vi "ConfigInstr.vi"(6 "InstrumentName":string, 7 "VisaRessIn":refnum<visa-resource-name>, 8 "error in (no error)":errorcluster caption="entrée d'erreur (pas d'erreur)", 9 "FirstClassInst":bool, 10 "Function":string, 11 "GenData In":refnum<class "SymphonyCCD.lvclass"> caption="DNL_LabVIEW Object in") -> (0 "error out":errorcluster caption="sortie d'erreur", 3 "GenData Out":refnum<class "SymphonyCCD.lvclass"> caption="DNL_LabVIEW Object out")   [LabVIEW 2019, in "SymphonyCCD.lvclass"]
uses:
  SymphonyCCD.lvclass
  C:/Programmes Labview/LabScanV1A/DevicesClass/BaseDevice/BaseDevice.lvclass
  SymphonyCCD_Func.ctl
  SymphonyCCD.lvclass/SymphonyCCD.ctl
  BaseDevice/BaseDevice.lvclass/BaseDevice.ctl
  BaseDevice/Accessor/SetShowInstrNm.vi
  BaseDevice/Accessor/SetSaveArrVarPar.vi
  BaseDevice/Accessor/SetInstrParam.vi
panel:
  in  "Class_Func":T1
  out "VisaRessOut":refnum<visa-resource-name>
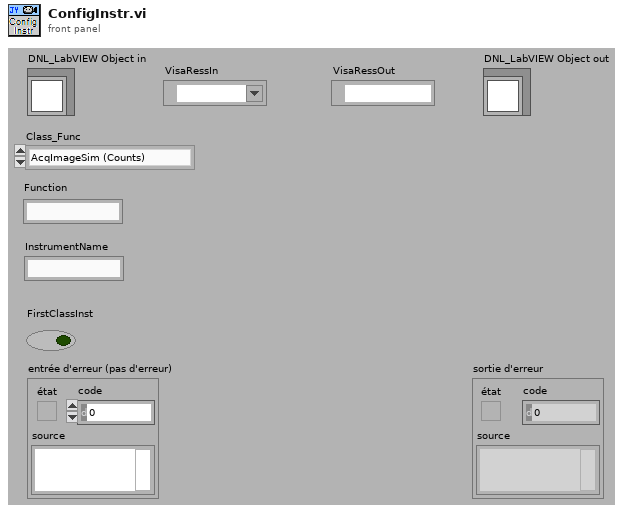
[diagram p1: front panel]
types:
  T1 = typedef "SymphonyCCD.lvclass/SymphonyCCD_Func.ctl" = enum16{"AcqImageSim (Counts)", "AcqImage (Counts)"}
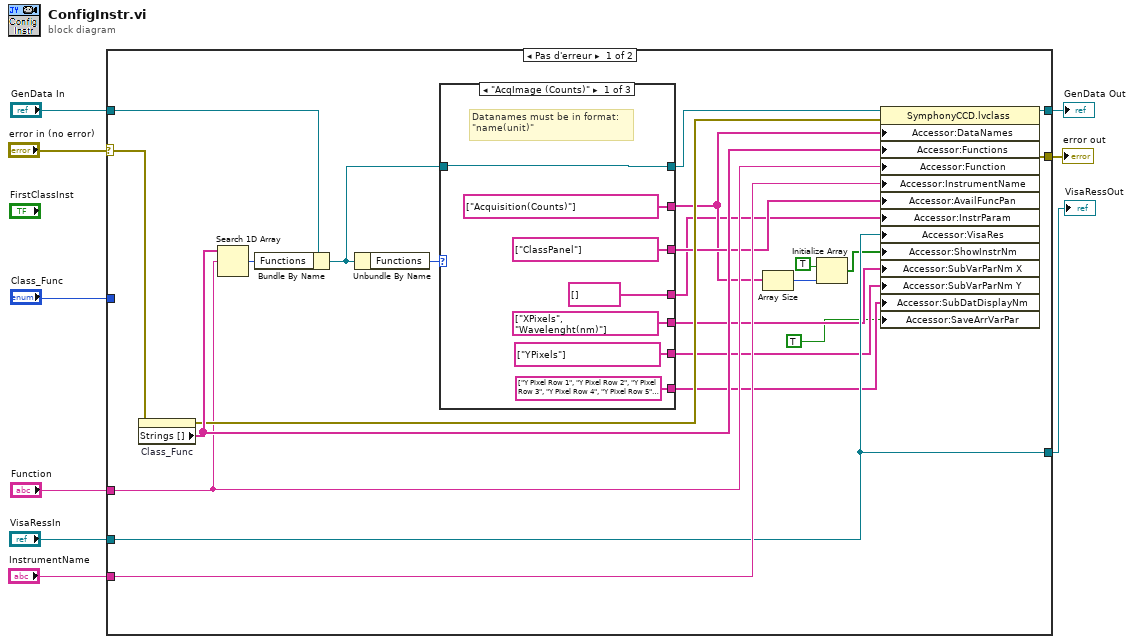
[diagram p0: block diagram]
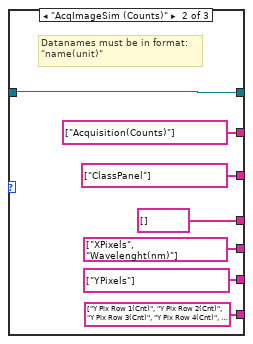
[diagram p2: hidden frame]
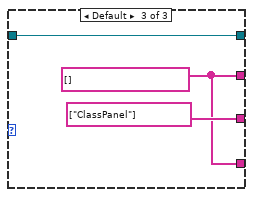
[diagram p3: hidden frame]
diagram:
  n1 = case shown="Pas d'erreur" "error in (no error)" {
    selector: "error in (no error)" -> [w26 w51]
    tunnel: [w32 w51] -> w8
    tunnel: "GenData In" -> [w27 w50]
    tunnel: [w31 w50] -> w6
    tunnel: "Class_Func" -> [_ _]
    tunnel: "Function" -> [w22 _]
    tunnel: "InstrumentName" -> [w21 _]
    tunnel: "VisaRessIn" -> [w19 _]
    tunnel: [w19 _] -> w1
    frame No Error {
      n2 = property on="Class_Func" class="Énum (strict)"(error in=w26) -> (error out=w25:errorcluster, "Strings []"=w29:string[])  [unwired: 1 in, 1 out]
      n3 = Search 1D Array(1D array=w29, element=w22) -> (index of element=w28:i32)  [unwired: 1 in]
      n4 = Bundle By Name(cluster=w27, "Functions"=w28) -> (w24:refnum<class "SymphonyCCD.lvclass">)
      n5 = Unbundle By Name(w24) -> ("Functions"=w30:T1)
      n6 = case shown="\"AcqImage (Counts)\"" w30 {
        tunnel: [string[] ["Acquisition(Counts)"] string[] ["Acquisition(Counts)"] w47] -> w16
        tunnel: w24 -> [w39 w46 w49]
        tunnel: [w39 w46 w49] -> w23
        tunnel: [string[] ["ClassPanel"] string[] ["ClassPanel"] string[] ["ClassPanel"]] -> w20
        tunnel: [string[] [] string[] [] w47] -> w14
        tunnel: [string[] ["XPixels", "Wavelenght(nm)"] string[] ["XPixels", "Wavelenght(nm)"] _] -> w13
        tunnel: [string[] ["YPixels"] string[] ["YPixels"] _] -> w12
        tunnel: [string[] ["Y Pixel Row 1", "Y Pixel Row 2", "Y Pixel Row 3", "Y Pixel Row 4", "Y Pixel Row 5", "Y Pixel Row 6", "Y Pixel Row 7", "Y Pixel Row 8", "Y Pixel Row 9", "Y Pixel Row 10", "Y Pixel Row 11", "Y Pixel Row 12", "Y Pixel Row 13", "Y Pixel Row 14", "Y Pixel Row 15", "Y Pixel Row 16", "Y Pixel Row 17", "Y Pixel Row 18", "Y Pixel Row 19", "Y Pixel Row 20", "Y Pixel Row 21", "Y Pixel Row 22", "Y Pixel Row 23", "Y Pixel Row 24", "Y Pixel Row 25", "Y Pixel Row 26", "Y Pixel Row 27", "Y Pixel Row 28", "Y Pixel Row 29", "Y Pixel Row 30", "Y Pixel Row 31", "Y Pixel Row 32", "Y Pixel Row 33", "Y Pixel Row 34", "Y Pixel Row 35", "Y Pixel Row 36", "Y Pixel Row 37", "Y Pixel Row 38", "Y Pixel Row 39", "Y Pixel Row 40", "Y Pixel Row 41", "Y Pixel Row 42", "Y Pixel Row 43", "Y Pixel Row 44", "Y Pixel Row 45", "Y Pixel Row 46", "Y Pixel Row 47", "Y Pixel Row 48", "Y Pixel Row 49", "Y Pixel Row 50", "Y Pixel Row 51", "Y Pixel Row 52", "Y Pixel Row 53", "Y Pixel Row 54", "Y Pixel Row 55", "Y Pixel Row 56", "Y Pixel Row 57", "Y Pixel Row 58", "Y Pixel Row 59", "Y Pixel Row 60", "Y Pixel Row 61", "Y Pixel Row 62", "Y Pixel Row 63", "Y Pixel Row 64", "Y Pixel Row 65", "Y Pixel Row 66", "Y Pixel Row 67", "Y Pixel Row 68", "Y Pixel Row 69", "Y Pixel Row 70", "Y Pixel Row 71", "Y Pixel Row 72", "Y Pixel Row 73", "Y Pixel Row 74", "Y Pixel Row 75", "Y Pixel Row 76", "Y Pixel Row 77", "Y Pixel Row 78", "Y Pixel Row 79", "Y Pixel Row 80", "Y Pixel Row 81", "Y Pixel Row 82", "Y Pixel Row 83", "Y Pixel Row 84", "Y Pixel Row 85", "Y Pixel Row 86", "Y Pixel Row 87", "Y Pixel Row 88", "Y Pixel Row 89", "Y Pixel Row 90", "Y Pixel Row 91", "Y Pixel Row 92", "Y Pixel Row 93", "Y Pixel Row 94", "Y Pixel Row 95", "Y Pixel Row 96", "Y Pixel Row 97", "Y Pixel Row 98", "Y Pixel Row 99", "Y Pixel Row 100", "Y Pixel Row 101", "Y Pixel Row 102", "Y Pixel Row 103", "Y Pixel Row 104", "Y Pixel Row 105", "Y Pixel Row 106", "Y Pixel Row 107", "Y Pixel Row 108", "Y Pixel Row 109", "Y Pixel Row 110", "Y Pixel Row 111", "Y Pixel Row 112", "Y Pixel Row 113", "Y Pixel Row 114", "Y Pixel Row 115", "Y Pixel Row 116", "Y Pixel Row 117", "Y Pixel Row 118", "Y Pixel Row 119", "Y Pixel Row 120", "Y Pixel Row 121", "Y Pixel Row 122", "Y Pixel Row 123", "Y Pixel Row 124", "Y Pixel Row 125", "Y Pixel Row 126", "Y Pixel Row 127", "Y Pixel Row 128", "Y Pixel Row 129", "Y Pixel Row 130", "Y Pixel Row 131", "Y Pixel Row 132", "Y Pixel Row 133", "Y Pixel Row 134", "Y Pixel Row 135", "Y Pixel Row 136", "Y Pixel Row 137", "Y Pixel Row 138", "Y Pixel Row 139", "Y Pixel Row 140", "Y Pixel Row 141", "Y Pixel Row 142", "Y Pixel Row 143", "Y Pixel Row 144", "Y Pixel Row 145", "Y Pixel Row 146", "Y Pixel Row 147", "Y Pixel Row 148", "Y Pixel Row 149", "Y Pixel Row 150", "Y Pixel Row 151", "Y Pixel Row 152", "Y Pixel Row 153", "Y Pixel Row 154", "Y Pixel Row 155", "Y Pixel Row 156", "Y Pixel Row 157", "Y Pixel Row 158", "Y Pixel Row 159", "Y Pixel Row 160", "Y Pixel Row 161", "Y Pixel Row 162", "Y Pixel Row 163", "Y Pixel Row 164", "Y Pixel Row 165", "Y Pixel Row 166", "Y Pixel Row 167", "Y Pixel Row 168", "Y Pixel Row 169", "Y Pixel Row 170", "Y Pixel Row 171", "Y Pixel Row 172", "Y Pixel Row 173", "Y Pixel Row 174", "Y Pixel Row 175", "Y Pixel Row 176", "Y Pixel Row 177", "Y Pixel Row 178", "Y Pixel Row 179", "Y Pixel Row 180", "Y Pixel Row 181", "Y Pixel Row 182", "Y Pixel Row 183", "Y Pixel Row 184", "Y Pixel Row 185", "Y Pixel Row 186", "Y Pixel Row 187", "Y Pixel Row 188", "Y Pixel Row 189", "Y Pixel Row 190", "Y Pixel Row 191", "Y Pixel Row 192", "Y Pixel Row 193", "Y Pixel Row 194", "Y Pixel Row 195", "Y Pixel Row 196", "Y Pixel Row 197", "Y Pixel Row 198", "Y Pixel Row 199", "Y Pixel Row 200", "Y Pixel Row 201", "Y Pixel Row 202", "Y Pixel Row 203", "Y Pixel Row 204", "Y Pixel Row 205", "Y Pixel Row 206", "Y Pixel Row 207", "Y Pixel Row 208", "Y Pixel Row 209", "Y Pixel Row 210", "Y Pixel Row 211", "Y Pixel Row 212", "Y Pixel Row 213", "Y Pixel Row 214", "Y Pixel Row 215", "Y Pixel Row 216", "Y Pixel Row 217", "Y Pixel Row 218", "Y Pixel Row 219", "Y Pixel Row 220", "Y Pixel Row 221", "Y Pixel Row 222", "Y Pixel Row 223", "Y Pixel Row 224", "Y Pixel Row 225", "Y Pixel Row 226", "Y Pixel Row 227", "Y Pixel Row 228", "Y Pixel Row 229", "Y Pixel Row 230", "Y Pixel Row 231", "Y Pixel Row 232", "Y Pixel Row 233", "Y Pixel Row 234", "Y Pixel Row 235", "Y Pixel Row 236", "Y Pixel Row 237", "Y Pixel Row 238", "Y Pixel Row 239", "Y Pixel Row 240", "Y Pixel Row 241", "Y Pixel Row 242", "Y Pixel Row 243", "Y Pixel Row 244", "Y Pixel Row 245", "Y Pixel Row 246", "Y Pixel Row 247", "Y Pixel Row 248", "Y Pixel Row 249", "Y Pixel Row 250", "Y Pixel Row 251", "Y Pixel Row 252", "Y Pixel Row 253", "Y Pixel Row 254", "Y Pixel Row 255", "Y Pixel Row 256"] string[] ["Y Pix Row 1(Cnt)", "Y Pix Row 2(Cnt)", "Y Pix Row 3(Cnt)", "Y Pix Row 4(Cnt)", "Y Pix Row 5(Cnt)", "Y Pix Row 6(Cnt)", "Y Pix Row 7(Cnt)", "Y Pix Row 8(Cnt)", "Y Pix Row 9(Cnt)", "Y Pix Row 10(Cnt)", "Y Pix Row 11(Cnt)", "Y Pix Row 12(Cnt)", "Y Pix Row 13(Cnt)", "Y Pix Row 14(Cnt)", "Y Pix Row 15(Cnt)", "Y Pix Row 16(Cnt)", "Y Pix Row 17(Cnt)", "Y Pix Row 18(Cnt)", "Y Pix Row 19(Cnt)", "Y Pix Row 20(Cnt)", "Y Pix Row 21(Cnt)", "Y Pix Row 22(Cnt)", "Y Pix Row 23(Cnt)", "Y Pix Row 24(Cnt)", "Y Pix Row 25(Cnt)", "Y Pix Row 26(Cnt)", "Y Pix Row 27(Cnt)", "Y Pix Row 28(Cnt)", "Y Pix Row 29(Cnt)", "Y Pix Row 30(Cnt)", "Y Pix Row 31(Cnt)", "Y Pix Row 32(Cnt)", "Y Pix Row 33(Cnt)", "Y Pix Row 34(Cnt)", "Y Pix Row 35(Cnt)", "Y Pix Row 36(Cnt)", "Y Pix Row 37(Cnt)", "Y Pix Row 38(Cnt)", "Y Pix Row 39(Cnt)", "Y Pix Row 40(Cnt)", "Y Pix Row 41(Cnt)", "Y Pix Row 42(Cnt)", "Y Pix Row 43(Cnt)", "Y Pix Row 44(Cnt)", "Y Pix Row 45(Cnt)", "Y Pix Row 46(Cnt)", "Y Pix Row 47(Cnt)", "Y Pix Row 48(Cnt)", "Y Pix Row 49(Cnt)", "Y Pix Row 50(Cnt)", "Y Pix Row 51(Cnt)", "Y Pix Row 52(Cnt)", "Y Pix Row 53(Cnt)", "Y Pix Row 54(Cnt)", "Y Pix Row 55(Cnt)", "Y Pix Row 56(Cnt)", "Y Pix Row 57(Cnt)", "Y Pix Row 58(Cnt)", "Y Pix Row 59(Cnt)", "Y Pix Row 60(Cnt)", "Y Pix Row 61(Cnt)", "Y Pix Row 62(Cnt)", "Y Pix Row 63(Cnt)", "Y Pix Row 64(Cnt)", "Y Pix Row 65(Cnt)", "Y Pix Row 66(Cnt)", "Y Pix Row 67(Cnt)", "Y Pix Row 68(Cnt)", "Y Pix Row 69(Cnt)", "Y Pix Row 70(Cnt)", "Y Pix Row 71(Cnt)", "Y Pix Row 72(Cnt)", "Y Pix Row 73(Cnt)", "Y Pix Row 74(Cnt)", "Y Pix Row 75(Cnt)", "Y Pix Row 76(Cnt)", "Y Pix Row 77(Cnt)", "Y Pix Row 78(Cnt)", "Y Pix Row 79(Cnt)", "Y Pix Row 80(Cnt)", "Y Pix Row 81(Cnt)", "Y Pix Row 82(Cnt)", "Y Pix Row 83(Cnt)", "Y Pix Row 84(Cnt)", "Y Pix Row 85(Cnt)", "Y Pix Row 86(Cnt)", "Y Pix Row 87(Cnt)", "Y Pix Row 88(Cnt)", "Y Pix Row 89(Cnt)", "Y Pix Row 90(Cnt)", "Y Pix Row 91(Cnt)", "Y Pix Row 92(Cnt)", "Y Pix Row 93(Cnt)", "Y Pix Row 94(Cnt)", "Y Pix Row 95(Cnt)", "Y Pix Row 96(Cnt)", "Y Pix Row 97(Cnt)", "Y Pix Row 98(Cnt)", "Y Pix Row 99(Cnt)", "Y Pix Row 100(Cnt)", "Y Pix Row 101(Cnt)", "Y Pix Row 102(Cnt)", "Y Pix Row 103(Cnt)", "Y Pix Row 104(Cnt)", "Y Pix Row 105(Cnt)", "Y Pix Row 106(Cnt)", "Y Pix Row 107(Cnt)", "Y Pix Row 108(Cnt)", "Y Pix Row 109(Cnt)", "Y Pix Row 110(Cnt)", "Y Pix Row 111(Cnt)", "Y Pix Row 112(Cnt)", "Y Pix Row 113(Cnt)", "Y Pix Row 114(Cnt)", "Y Pix Row 115(Cnt)", "Y Pix Row 116(Cnt)", "Y Pix Row 117(Cnt)", "Y Pix Row 118(Cnt)", "Y Pix Row 119(Cnt)", "Y Pix Row 120(Cnt)", "Y Pix Row 121(Cnt)", "Y Pix Row 122(Cnt)", "Y Pix Row 123(Cnt)", "Y Pix Row 124(Cnt)", "Y Pix Row 125(Cnt)", "Y Pix Row 126(Cnt)", "Y Pix Row 127(Cnt)", "Y Pix Row 128(Cnt)", "Y Pix Row 129(Cnt)", "Y Pix Row 130(Cnt)", "Y Pix Row 131(Cnt)", "Y Pix Row 132(Cnt)", "Y Pix Row 133(Cnt)", "Y Pix Row 134(Cnt)", "Y Pix Row 135(Cnt)", "Y Pix Row 136(Cnt)", "Y Pix Row 137(Cnt)", "Y Pix Row 138(Cnt)", "Y Pix Row 139(Cnt)", "Y Pix Row 140(Cnt)", "Y Pix Row 141(Cnt)", "Y Pix Row 142(Cnt)", "Y Pix Row 143(Cnt)", "Y Pix Row 144(Cnt)", "Y Pix Row 145(Cnt)", "Y Pix Row 146(Cnt)", "Y Pix Row 147(Cnt)", "Y Pix Row 148(Cnt)", "Y Pix Row 149(Cnt)", "Y Pix Row 150(Cnt)", "Y Pix Row 151(Cnt)", "Y Pix Row 152(Cnt)", "Y Pix Row 153(Cnt)", "Y Pix Row 154(Cnt)", "Y Pix Row 155(Cnt)", "Y Pix Row 156(Cnt)", "Y Pix Row 157(Cnt)", "Y Pix Row 158(Cnt)", "Y Pix Row 159(Cnt)", "Y Pix Row 160(Cnt)", "Y Pix Row 161(Cnt)", "Y Pix Row 162(Cnt)", "Y Pix Row 163(Cnt)", "Y Pix Row 164(Cnt)", "Y Pix Row 165(Cnt)", "Y Pix Row 166(Cnt)", "Y Pix Row 167(Cnt)", "Y Pix Row 168(Cnt)", "Y Pix Row 169(Cnt)", "Y Pix Row 170(Cnt)", "Y Pix Row 171(Cnt)", "Y Pix Row 172(Cnt)", "Y Pix Row 173(Cnt)", "Y Pix Row 174(Cnt)", "Y Pix Row 175(Cnt)", "Y Pix Row 176(Cnt)", "Y Pix Row 177(Cnt)", "Y Pix Row 178(Cnt)", "Y Pix Row 179(Cnt)", "Y Pix Row 180(Cnt)", "Y Pix Row 181(Cnt)", "Y Pix Row 182(Cnt)", "Y Pix Row 183(Cnt)", "Y Pix Row 184(Cnt)", "Y Pix Row 185(Cnt)", "Y Pix Row 186(Cnt)", "Y Pix Row 187(Cnt)", "Y Pix Row 188(Cnt)", "Y Pix Row 189(Cnt)", "Y Pix Row 190(Cnt)", "Y Pix Row 191(Cnt)", "Y Pix Row 192(Cnt)", "Y Pix Row 193(Cnt)", "Y Pix Row 194(Cnt)", "Y Pix Row 195(Cnt)", "Y Pix Row 196(Cnt)", "Y Pix Row 197(Cnt)", "Y Pix Row 198(Cnt)", "Y Pix Row 199(Cnt)", "Y Pix Row 200(Cnt)", "Y Pix Row 201(Cnt)", "Y Pix Row 202(Cnt)", "Y Pix Row 203(Cnt)", "Y Pix Row 204(Cnt)", "Y Pix Row 205(Cnt)", "Y Pix Row 206(Cnt)", "Y Pix Row 207(Cnt)", "Y Pix Row 208(Cnt)", "Y Pix Row 209(Cnt)", "Y Pix Row 210(Cnt)", "Y Pix Row 211(Cnt)", "Y Pix Row 212(Cnt)", "Y Pix Row 213(Cnt)", "Y Pix Row 214(Cnt)", "Y Pix Row 215(Cnt)", "Y Pix Row 216(Cnt)", "Y Pix Row 217(Cnt)", "Y Pix Row 218(Cnt)", "Y Pix Row 219(Cnt)", "Y Pix Row 220(Cnt)", "Y Pix Row 221(Cnt)", "Y Pix Row 222(Cnt)", "Y Pix Row 223(Cnt)", "Y Pix Row 224(Cnt)", "Y Pix Row 225(Cnt)", "Y Pix Row 226(Cnt)", "Y Pix Row 227(Cnt)", "Y Pix Row 228(Cnt)", "Y Pix Row 229(Cnt)", "Y Pix Row 230(Cnt)", "Y Pix Row 231(Cnt)", "Y Pix Row 232(Cnt)", "Y Pix Row 233(Cnt)", "Y Pix Row 234(Cnt)", "Y Pix Row 235(Cnt)", "Y Pix Row 236(Cnt)", "Y Pix Row 237(Cnt)", "Y Pix Row 238(Cnt)", "Y Pix Row 239(Cnt)", "Y Pix Row 240(Cnt)", "Y Pix Row 241(Cnt)", "Y Pix Row 242(Cnt)", "Y Pix Row 243(Cnt)", "Y Pix Row 244(Cnt)", "Y Pix Row 245(Cnt)", "Y Pix Row 246(Cnt)", "Y Pix Row 247(Cnt)", "Y Pix Row 248(Cnt)", "Y Pix Row 249(Cnt)", "Y Pix Row 250(Cnt)", "Y Pix Row 251(Cnt)", "Y Pix Row 252(Cnt)", "Y Pix Row 253(Cnt)", "Y Pix Row 254(Cnt)", "Y Pix Row 255(Cnt)", "Y Pix Row 256(Cnt)"] _] -> w11
        frame "AcqImage (Counts)" {
          # "Datanames must be in format:\n\"name(unit)\""
        }
        frame "AcqImageSim (Counts)" {
          # "Datanames must be in format:\n\"name(unit)\""
        }
        frame Default {
          w47 = string[] []
        }
      }
      n7 = Array Size(array=w16) -> (size(s)=w18:i32)
      n8 = Initialize Array(TRUE, w18) -> (w15:bool[])
      n9 = property class="SymphonyCCD.lvclass"(reference=w23, error in=w25, "Accessor:DataNames"=w16, "Accessor:Functions"=w29, "Accessor:Function"=w22, "Accessor:InstrumentName"=w21, "Accessor:AvailFuncPan"=w20, "Accessor:InstrParam"=w14, "Accessor:VisaRes"=w19, "Accessor:ShowInstrNm"=w15, "Accessor:SubVarParNm X"=w13, "Accessor:SubVarParNm Y"=w12, "Accessor:SubDatDisplayNm"=w11, "Accessor:SaveArrVarPar"=TRUE ("SaveArrVarPar")) -> (reference out=w31:refnum<class "SymphonyCCD.lvclass">, error out=w32:errorcluster)
    }
    frame Error {
    }
  }
  "error out" <- w8
  "GenData Out" <- w6
  "VisaRessOut" <- w1
